vi "Layout - Load Modules into Subpanels.vi"(7 "SubPanels - in":T1, 8 "error in (no error)":errorcluster, 10 "Module Names":string[](array[string]), 11 "SubPanel Names":string[](array[string])) -> (0 "error out":errorcluster, 5 "SubPanels --out":T1)   [LabVIEW 2022 SP3, in "UI Manager.lvlib"]
doc: "Loads the DQMH modules in <b>Module Names</b> into the <b>Subpanel References</b>.\n\n____\nHAMPEL SOFTWARE ENGINEERING v2.6.0 (2023-12-19 10:54)"
uses:
  UI Manager.lvlib
  Libraries/hse-libraries/Source/hse-ui/hse-ui.lvlib
  Libraries/hse-libraries/Source/hse-dqmh/hse-dqmh-dynamicrequesters.lvlib
  Libraries/hse-libraries/Source/hse-application/hse-application.lvclass
  <vilib>/Utility/miscctls.llb/LVMapReplaceAction.ctl
  SubPanels--map.ctl
  SubPnl Map References--cluster.ctl
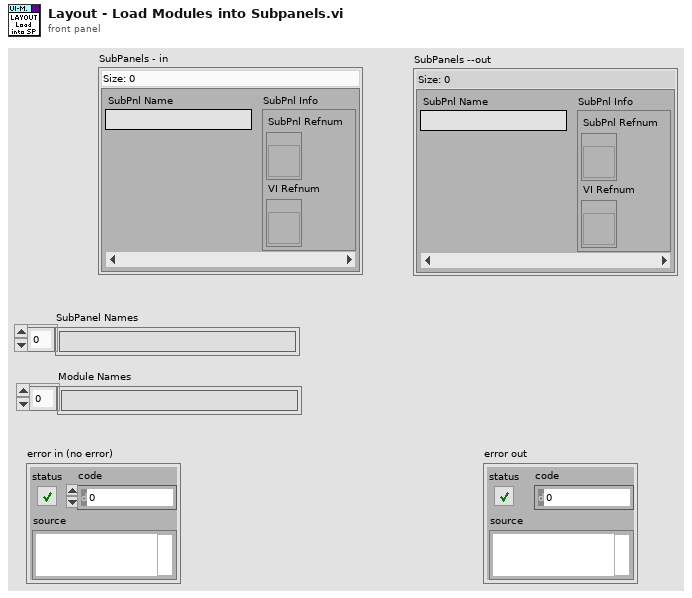
[diagram p1: front panel]
types:
  T1 = typedef "UI Manager.lvlib/SubPanels--map.ctl" = map{string, T2}
  T2 = typedef "UI Manager.lvlib/SubPnl Map References--cluster.ctl" = cluster{"SubPnl Refnum":refnum<vi>, "VI Refnum":refnum<vi>}
  T3 = typedef "LVMapReplaceAction.ctl" = enum32{"Modify Entry only if found", "Add or Modify Entry", "Delete Entry"}
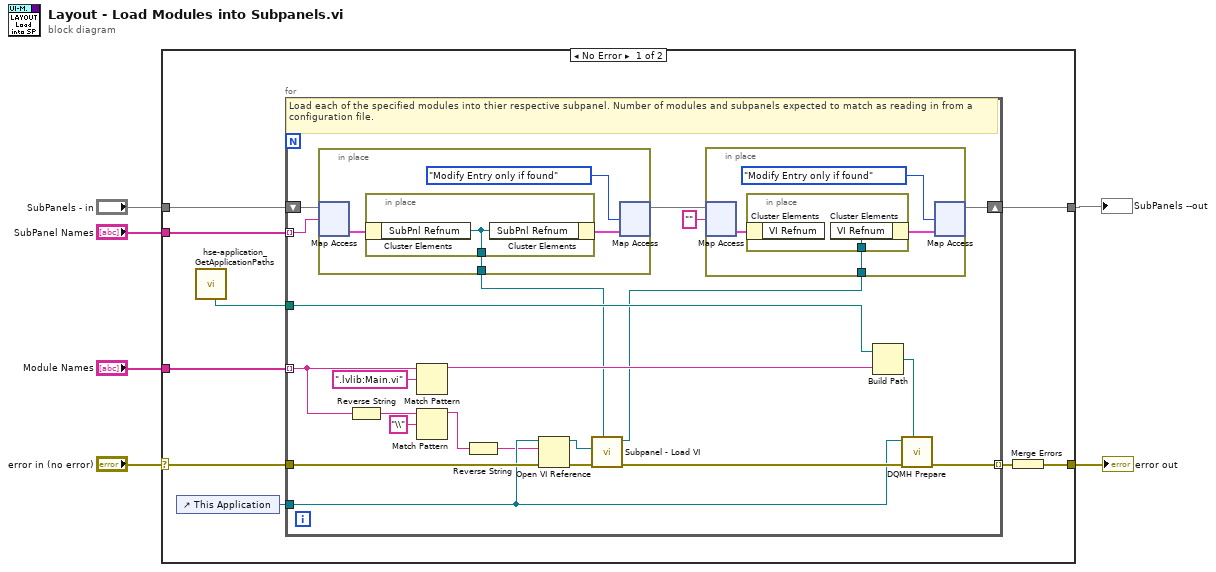
[diagram p0: block diagram]
diagram:
  n1 = case shown="No Error" "error in (no error)" {
    selector: "error in (no error)" -> [w14 w49]
    tunnel: "Module Names" -> [w11 _]
    tunnel: [w15 w49] -> w4
    tunnel: "SubPanel Names" -> [w12 _]
    tunnel: "SubPanels - in" -> [w8 w48]
    tunnel: [w7 w48] -> w1
    frame No Error {
      n2 = control-ref of="This Application"() -> (w10:refnum<vi>)
      n3 = call "hse-application_GetApplicationPaths.vi"() -> ("Application Base Path"=w9:path)  [unwired: 5 in, 6 out]
      n4 = for {
        tunnel: w14 -> [w36]
        tunnel: [w33] -> w13 mode=indexing
        tunnel: w12 -> [w20] mode=indexing
        tunnel: w11 -> [w24] mode=indexing
        tunnel: w10 -> [w30]
        tunnel: w9 -> [w32]
        shift-right: [w18] -> w7
        shift-left: w8 -> [w22]
        # "Load each of the specified modules into thier respective subpanel. Number of modules and subpanels expected to match as reading in from a configuration file."
        n5 = in-place {
          in-place-border: [w45] -> w21
          n6 = in-place-map #1(w22, w20) -> (w46:T2)  [unwired: 1 in, 1 out]
          n7 = in-place {
            in-place-border: [w47] -> w45
            n8 = in-place-cluster #2(w46) -> ("SubPnl Refnum"=w47:refnum<vi>)
            n9 = in-place-cluster #2("SubPnl Refnum"=w47) -> (w43:T2)
          }
          n10 = in-place-map #1(w43, LVMapReplaceAction."Modify Entry only if found" ("action")) -> (w19:T1)  [unwired: 2 out]
        }
        n11 = Reverse String(1:w24) -> (0:w25:string)
        n12 = Match Pattern(string=w24, regular expression=".lvlib:Main.vi") -> (before substring=w23:string)  [unwired: 1 in, 3 out]
        n13 = Match Pattern(string=w25, regular expression="\\") -> (before substring=w28:string)  [unwired: 1 in, 3 out]
        n14 = Reverse String(1:w28) -> (0:w27:string)
        n15 = Open VI Reference(application reference (local)=w30, vi path=w27, error in (no error)=w36) -> (vi reference=w37:refnum<vi>, error out=w35:errorcluster)  [unwired: 3 in]
        n16 = call "Subpanel - Load VI.vi"("SubPanel in"=w21, "error in (no error)"=w35, "VI Reference"=w37) -> ("error out"=w34:errorcluster, "Subpanel VI Ref OUT"=w17:refnum<vi>)  [unwired: 6 in, 1 out]
        n17 = in-place {
          in-place-border: w17 -> [w38]
          n18 = in-place-map #3(w19, "" ("String")) -> (w39:T2)  [unwired: 1 in, 1 out]
          n19 = in-place {
            in-place-border: w38 -> [w42]
            n20 = in-place-cluster #4(w39) -> ()  [unwired: 1 out]
            n21 = in-place-cluster #4("VI Refnum"=w42) -> (w40:T2)
          }
          n22 = in-place-map #3(w40, LVMapReplaceAction."Modify Entry only if found" ("action")) -> (w18:T1)  [unwired: 2 out]
        }
        n23 = Build Path(base path=w32, name or relative path=w23) -> (appended path=w31:path)
        n24 = call "DQMH Prepare.vi"("Module Disk Path"=w31, "error in (no error)"=w34, "Application reference"=w30) -> ("error out"=w33:errorcluster)  [unwired: 8 in]
      }
      n25 = Merge Errors(w13) -> (w15:errorcluster)
    }
    frame Error {
    }
  }
  "error out" <- w4
  "SubPanels --out" <- w1
